vi "octave_check_exit_code.vi"(8 "error in":errorcluster, 11 "instance handle in":u32[](array[numeric])) -> (0 "error out":errorcluster, 1 "exited":bool, 2 "running":bool, 3 "instance handle out":u32[](array[numeric]), 4 "exit code":i32)   [LabVIEW 2011]
doc: "This VI checks process instance status. It signalizes if Octave is still running or already returned exit code. In that case exit code it returned.\nIf no process instance handle is connected, last one from global variable is used or new instance handle is stored to it.\nProcess instance handle can be automatically closed if process has exited."
uses:
  octave_var.vi
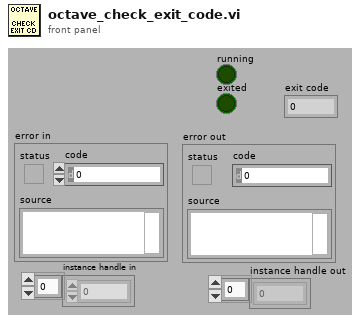
[diagram p1: front panel]
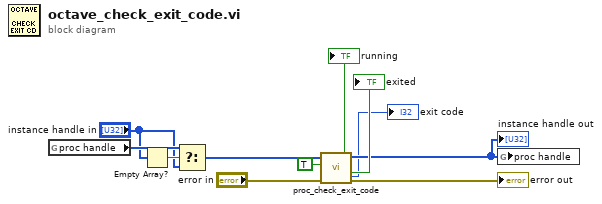
[diagram p0: block diagram]
diagram:
  n1 = global read "octave_var.vi" "proc handle"() -> (w10:u32[])
  n2 = Empty Array?(array="instance handle in") -> (empty?=w9:bool)
  n3 = Select(t=w10, s=w9, f="instance handle in") -> (s? t:f=w7:u32[])
  n4 = call "proc_check_exit_code.vi"("error in"="error in", "ignore error"=TRUE, "instance handle in"=w7) -> ("error out"=→"error out":errorcluster, "exited"=→"exited":bool, "running"=→"running":bool, "instance handle out"=w4:u32[], "exit code"=→"exit code":i32)  [unwired: 4 in]
  "instance handle out" <- w4
  n5 = global write "octave_var.vi" "proc handle"(w4) -> ()
